vi "Turret Initialization.vi"(10 "DIO Channels":cluster{"Turret Encoder":T5, "Hood Encoder":T5}, 11 "Motor CAN IDs":T6={"Shooter Left"=12, "Shooter Right"=13, "Turret"=14, "Hood"=14}) -> (1 "Hood":T1, 2 "Turret":T1, 3 "Shooter":T1)   [LabVIEW 2019]
uses:
  <vilib>/Rock Robotics/SystemInterfaces/DutyCycle/FPGA_DutyCycleDevRef.ctl
  <vilib>/Rock Robotics/SystemInterfaces/DutyCycle/FPGA_DutyCycleIndex.ctl
  <vilib>/Rock Robotics/WPI/MotorControl/WPI_MotorControlDeviceRef.ctl
  <vilib>/Rock Robotics/WPI/MotorControl/WPI_MotorControlType.ctl
  <vilib>/Rock Robotics/SystemInterfaces/DIO/FPGA_DIOPWMChannel.ctl
  <vilib>/Rock Robotics/WPI/PWM/WPI_PWMDeadband.ctl
  <vilib>/Rock Robotics/SystemInterfaces/DIO/FPGA_DIOChannel.ctl
  <vilib>/Rock Robotics/WPI/ThirdParty/REV Robotics/SPARK MAX/Typedef/Spark MAX Motor Type.ctl
  <vilib>/Rock Robotics/WPI/ThirdParty/REV Robotics/SPARK MAX/Typedef/Spark MAX Idle Mode.ctl
  Turret Published Globals.vi
  <vilib>/Rock Robotics/WPI/Counter/WPI_CounterDigitalInputToDigitalSource.vi
panel:
  out "Hood Encoder":T7
  out "Turret Encoder":T7
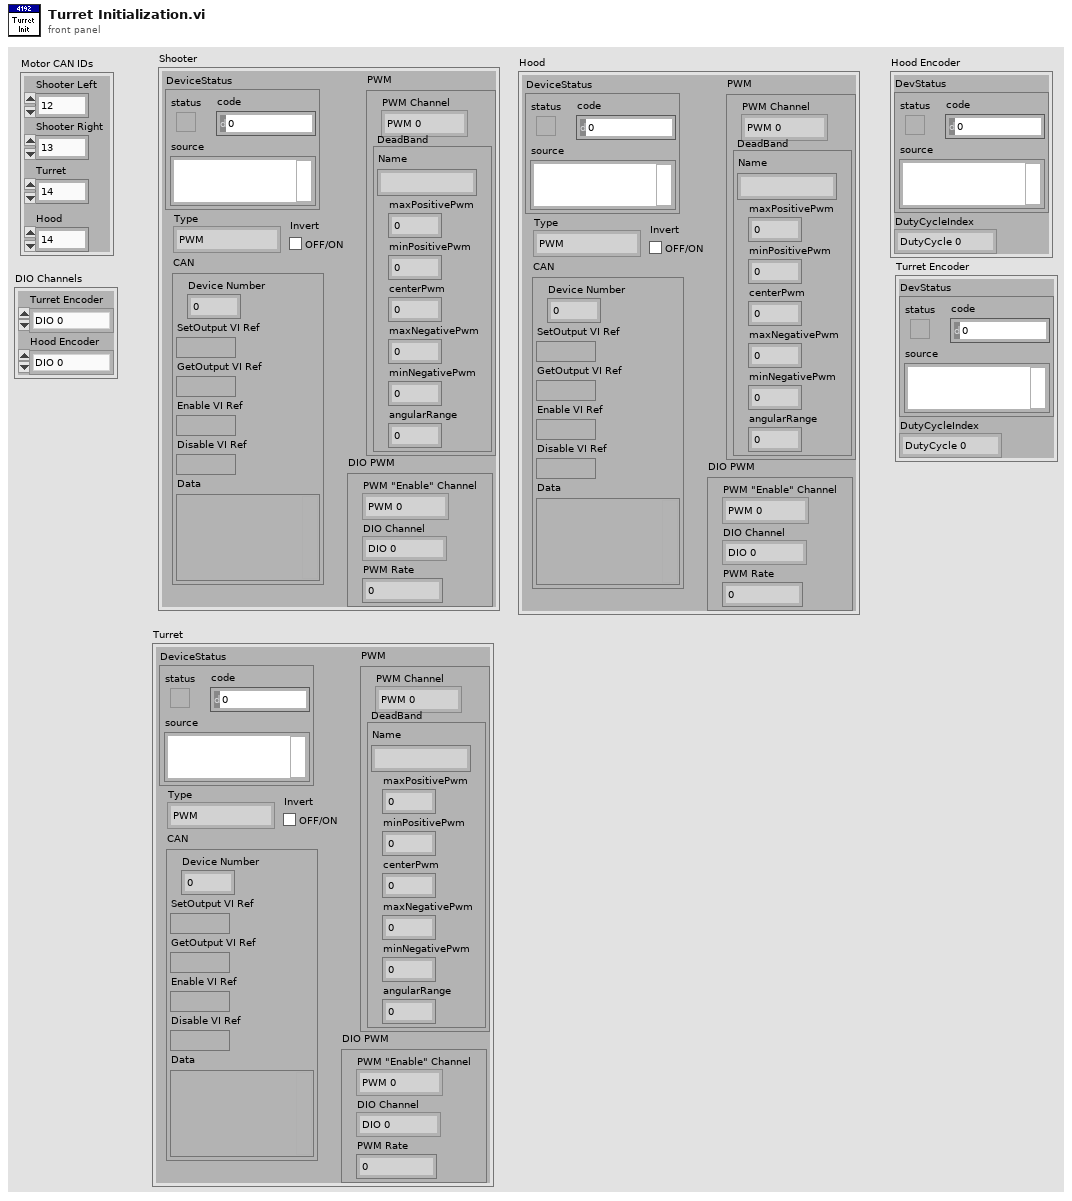
[diagram p1: front panel]
types:
  T1 = typedef "WPI_MotorControlDeviceRef.ctl" = cluster{"DeviceStatus":errorcluster, "Type":T2, "PWM":cluster{"PWM Channel":T3, "DeadBand":T4}, "CAN":cluster{"Device Number":u8, "SetOutput VI Ref":variant, "GetOutput VI Ref":variant, "Enable VI Ref":variant, "Disable VI Ref":variant, "Data":variant}, "Invert":bool, "DIO PWM":cluster{"PWM \"Enable\" Channel":T3, "DIOChannel":T5, "PWM Rate":dbl}}
  T2 = typedef "WPI_MotorControlType.ctl" = enum16{"PWM", "CAN", "DIO PWM"}
  T3 = typedef "FPGA_DIOPWMChannel.ctl" = enum8{"PWM 0", "PWM 1", "PWM 2", "PWM 3", "PWM 4", "PWM 5", "PWM 6", "PWM 7", "PWM 8", "PWM 9", "PWM MXP 0", "PWM MXP 1", "PWM MXP 2", "PWM MXP 3", "PWM MXP 4", "PWM MXP 5", "PWM MXP 6", "PWM MXP 7", "PWM MXP 8", "PWM MXP 9", "Invalid"}
  T4 = typedef "WPI_PWMDeadband.ctl" = cluster{"Name":string, "maxPositivePwm":i32, "minPositivePwm":i32, "centerPwm":i32, "maxNegativePwm":i32, "minNegativePwm":i32, "angularRange":u16}
  T5 = typedef "FPGA_DIOChannel.ctl" = enum8{"DIO 0", "DIO 1", "DIO 2", "DIO 3", "DIO 4", "DIO 5", "DIO 6", "DIO 7", "DIO 8", "DIO 9", "DIO MXP 0", "DIO MXP 1", "DIO MXP 2", "DIO MXP 3", "DIO MXP 4", "DIO MXP 5", "DIO MXP 6", "DIO MXP 7", "DIO MXP 8", "DIO MXP 9", "DIO MXP 10", "DIO MXP 11", "DIO MXP 12", "DIO MXP 13", "DIO MXP 14", "DIO MXP 15", "SPI Port CS1", "SPI Port CS2", "SPI Port CS3", "SPI Port MISO", "SPI Port MOSI", "Invalid"}
  T6 = cluster{"Shooter Left":u8, "Shooter Right":u8, "Turret":u8, "Hood":u8}
  T7 = typedef "FPGA_DutyCycleDevRef.ctl" = cluster{"DevStatus":errorcluster, "DutyCycleIndex":T8}
  T8 = typedef "FPGA_DutyCycleIndex.ctl" = enum8{"DutyCycle 0", "DutyCycle 1", "DutyCycle 2", "DutyCycle 3", "DutyCycle 4", "DutyCycle 5", "DutyCycle 6", "DutyCycle 7", "Invalid"}
  T9 = typedef "Spark MAX Idle Mode.ctl" = enum16{"Coast", "Brake"}
  T10 = typedef "Spark MAX Motor Type.ctl" = enum16{"Brushed", "Brushless"}
  T11 = typedef "WPI_DigitalInputDevRef.ctl" = cluster{"DevStatus":errorcluster, "DIO Channel":T5}
  T12 = typedef "FPGA_CounterEncoderSourceConvertionLVSourceType.ctl" = cluster{"DevStatus":errorcluster, "AnalogTriggerMode?":bool, "DigitalMode":cluster{"DIO Channel":T13}, "AnalogTriggerMode":cluster{"AnalogTriggerIndex":T14, "OutputType":T15}}
  T13 = typedef "FPGA_DIODigitalSourceChannel.ctl" = enum8{"DIO 0", "DIO 1", "DIO 2", "DIO 3", "DIO 4", "DIO 5", "DIO 6", "DIO 7", "DIO 8", "DIO 9", "DIO MXP 0", "DIO MXP 1", "DIO MXP 2", "DIO MXP 3", "DIO MXP 4", "DIO MXP 5", "DIO MXP 6", "DIO MXP 7", "DIO MXP 8", "DIO MXP 9", "DIO MXP 10", "DIO MXP 11", "DIO MXP 12", "DIO MXP 13", "DIO MXP 14", "DIO MXP 15", "SPI Port CS1", "SPI Port CS2", "SPI Port CS3", "SPI Port MISO", "SPI Port MOSI", "Disabled"}
  T14 = typedef "FPGA_AnalogTriggerIndex.ctl" = enum8{"Trig 0", "Trig 1", "Trig 2", "Trig 3", "Trig 4", "Trig 5", "Trig 6", "Trig 7", "Invalid"}
  T15 = typedef "FPGA_AnalogTriggerOutType.ctl" = enum16{"InWindow", "TriggerState", "Rising", "Falling"}
  T16 = cluster{"Shooter Up To Speed?":bool, "Aligned With Target?":bool, "Hood at Angle?":bool, "Shooting?":bool, "Hood Angle":dbl, "Turret Angle":dbl, "Shooter Velocity":dbl}
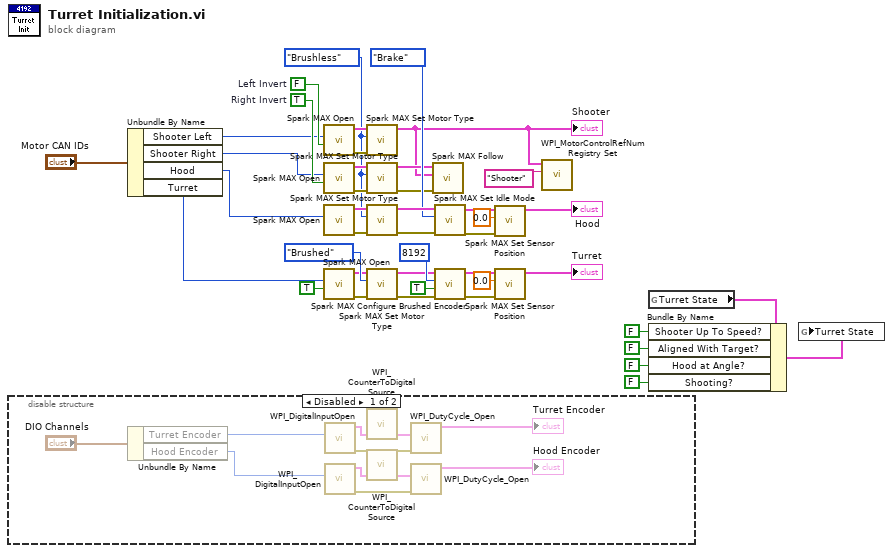
[diagram p0: block diagram]
diagram:
  w43 = FALSE  # Left Invert
  w42 = TRUE  # Right Invert
  w30 = Spark_MAX_Motor_Type."Brushless" ("Motor Type")
  n1 = disable-structure shown="Disabled" {
    frame Disabled {
      n2 = Unbundle By Name("DIO Channels") -> ("Turret Encoder"=w49:T5, "Hood Encoder"=w54:T5)
      n3 = call <vilib>:"WPI_DigitalInputOpen.vi"("DIO Channel"=w49) -> ("error out"=w45:errorcluster, "DigitalInputDevRef"=w46:T11)  [unwired: 9 in]
      n4 = call <vilib>:"WPI_DigitalInputOpen.vi"("DIO Channel"=w54) -> ("error out"=w52:errorcluster, "DigitalInputDevRef"=w53:T11)  [unwired: 9 in]
      n5 = call-poly <vilib>:"WPI_CounterToDigitalSource.vi"("DigitalInputDevRef"=w46) -> ("Digital Source"=w47:T12)  [unwired: 6 in]
      n6 = call-poly <vilib>:"WPI_CounterToDigitalSource.vi"("DigitalInputDevRef"=w53) -> ("Digital Source"=w51:T12)  [unwired: 6 in]
      n7 = call <vilib>:"WPI_DutyCycle_Open.vi"("error in (no error)"=w45, "Source"=w47) -> ("DutyCycleDevRef"=→"Turret Encoder":T7)  [unwired: 8 in, 1 out]
      n8 = call <vilib>:"WPI_DutyCycle_Open.vi"("error in (no error)"=w52, "Source"=w51) -> ("DutyCycleDevRef"=→"Hood Encoder":T7)  [unwired: 8 in, 1 out]
    }
    frame Enabled {
    }
  }
  n9 = Unbundle By Name("Motor CAN IDs") -> ("Shooter Left"=w33:u8, "Shooter Right"=w34:u8, "Hood"=w28:u8, "Turret"=w27:u8)
  n10 = call <vilib>:"Spark MAX Open.vi"("Invert"=w43, "Device Number"=w33) -> ("error out"=w38:errorcluster, "MotorControlDeviceRef"=w39:T1)  [unwired: 8 in]
  n11 = call <vilib>:"Spark MAX Open.vi"("Invert"=w42, "Device Number"=w34) -> ("error out"=w40:errorcluster, "MotorControlDeviceRef"=w41:T1)  [unwired: 8 in]
  n12 = call <vilib>:"Spark MAX Open.vi"("Device Number"=w28) -> ("error out"=w29:errorcluster, "MotorControlDeviceRef"=w31:T1)  [unwired: 9 in]
  n13 = call <vilib>:"Spark MAX Open.vi"("Invert"=TRUE, "Device Number"=w27) -> ("error out"=w35:errorcluster, "MotorControlDeviceRef"=w36:T1)  [unwired: 8 in]
  n14 = call <vilib>:"Spark MAX Set Motor Type.vi"("error in (no error)"=w38, "Motor Type"=w30, "MotorControlDevRef"=w39) -> ("MotorControlDeviceRef"=w2:T1)  [unwired: 7 in, 1 out]
  "Shooter" <- w2
  n15 = call <vilib>:"Spark MAX Set Motor Type.vi"("error in (no error)"=w40, "Motor Type"=w30, "MotorControlDevRef"=w41) -> ("error out"=w3:errorcluster, "MotorControlDeviceRef"=w4:T1)  [unwired: 7 in]
  n16 = call <vilib>:"Spark MAX Set Motor Type.vi"("error in (no error)"=w29, "Motor Type"=w30, "MotorControlDevRef"=w31) -> ("error out"=w25:errorcluster, "MotorControlDeviceRef"=w26:T1)  [unwired: 7 in]
  n17 = call <vilib>:"Spark MAX Set Motor Type.vi"("error in (no error)"=w35, "Motor Type"=Spark_MAX_Motor_Type."Brushed", "MotorControlDevRef"=w36) -> ("error out"=w23:errorcluster, "MotorControlDeviceRef"=w21:T1)  [unwired: 7 in]
  n18 = call <vilib>:"Spark MAX Follow.vi"("error in (no error)"=w3, "Master Controller"=w2, "MotorControlDeviceRef"=w4) -> ()  [unwired: 7 in, 2 out]
  n19 = call <vilib>:"Spark MAX Set Idle Mode.vi"("error in (no error)"=w25, "Idle Mode"=Spark_MAX_Idle_Mode."Brake", "MotorControlDeviceRef in"=w26) -> ("error out"=w18:errorcluster, "MotorControlDeviceRef out"=w20:T1)  [unwired: 7 in]
  n20 = call <vilib>:"Spark MAX Configure Brushed Encoder.vi"("error in (no error)"=w23, "Inverted (F)"=TRUE, "Cycles per Revolution (4096)"=u32 8192, "MotorControlDeviceRef in"=w21) -> ("error out"=w13:errorcluster, "MotorControlDeviceRef"=w16:T1)  [unwired: 6 in]
  n21 = call <vilib>:"Spark MAX Set Sensor Position.vi"("error in"=w18, "Position"=0.0, "MotorControlDeviceRef"=w20) -> ("MotorControlDeviceRef"=→"Hood":T1)  [unwired: 7 in, 1 out]
  n22 = call <vilib>:"Spark MAX Set Sensor Position.vi"("error in"=w13, "Position"=0.0, "MotorControlDeviceRef"=w16) -> ("MotorControlDeviceRef"=→"Turret":T1)  [unwired: 7 in, 1 out]
  n23 = call <vilib>:"WPI_MotorControlRefNum Registry Set.vi"("refnum name"="Shooter", "MotorControlDevRef"=w2) -> ()  [unwired: 8 in, 2 out]
  n24 = global read "Turret Published Globals.vi" "Turret State"() -> (w9:T16)
  n25 = Bundle By Name(cluster=w9, "Shooter Up To Speed?"=FALSE, "Aligned With Target?"=FALSE, "Hood at Angle?"=FALSE, "Shooting?"=FALSE) -> (w10:T16)
  n26 = global write "Turret Published Globals.vi" "Turret State"(w10) -> ()
